vi "UI_Elmts_Reads[Labels].vi"(8 "error in (no error)":errorcluster, 10 "Elmts Labels":string[](array[string]), 11 "UI_Actor in":refnum<class "UI_Actor.lvclass">) -> (0 "error out":errorcluster, 1 "Founds":bool[](array[boolean]), 2 "Values":variant[](array[variant]), 3 "UI_Actor out":refnum<class "UI_Actor.lvclass">)   [LabVIEW 2020, in "UI_Actor.lvlib" / "UI_Actor.lvclass"]
uses:
  UI_Actor.lvclass
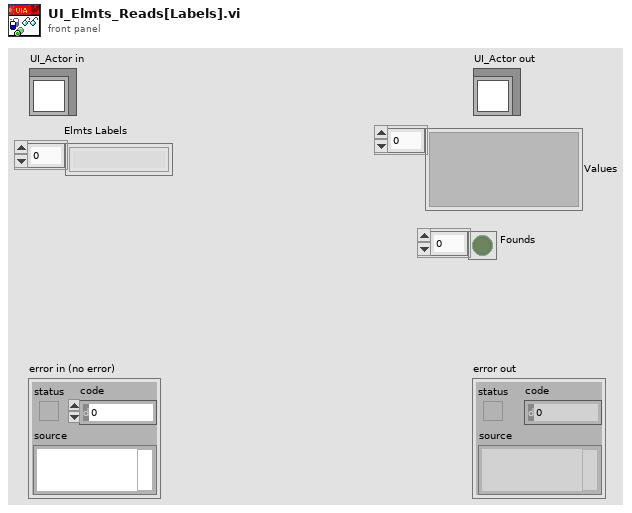
[diagram p1: front panel]
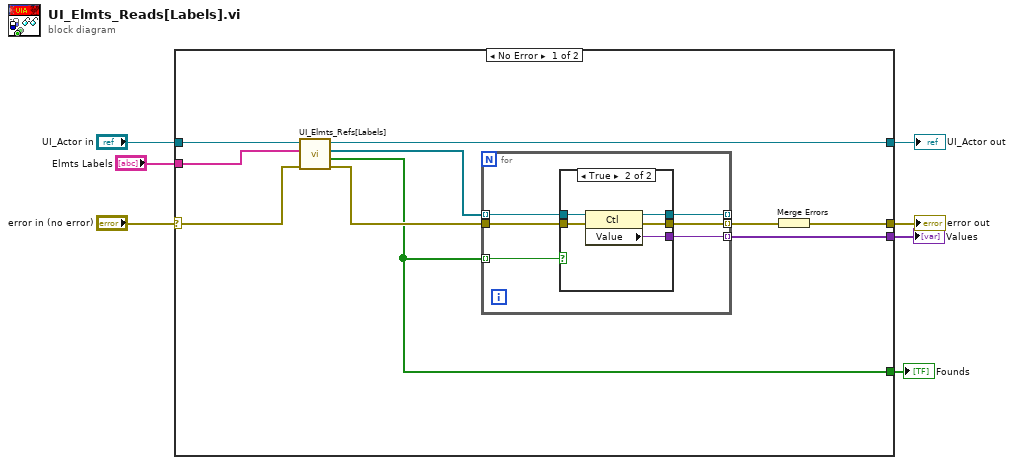
[diagram p0: block diagram]
diagram:
  n1 = case shown="No Error" "error in (no error)" {
    selector: "error in (no error)" -> [w12 w32]
    tunnel: [w14 w32] -> w6
    tunnel: [w16 w31] -> w4
    tunnel: "UI_Actor in" -> [w17 w31]
    tunnel: "Elmts Labels" -> [w15 _]
    tunnel: [w13 _] -> w1
    tunnel: [w8 _] -> w2
    frame No Error {
      n2 = call "UI_Elmts_Refs[Labels].vi"("error in (no error)"=w12, "Elmts Labels"=w15, "UI_Actor in"=w17) -> ("error out"=w11:errorcluster, "Founds"=w8:bool[], "Refs"=w10:refnum<vi>[], "UI_Actor out"=w16:refnum<class "UI_Actor.lvclass">)  [unwired: 5 in]
      n3 = for {
        tunnel: w10 -> [w21] mode=indexing
        tunnel: [w20] -> w13 mode=indexing
        tunnel: [w19] -> _ mode=indexing
        tunnel: w11 -> [w23]
        tunnel: [w22] -> w9 mode=indexing
        tunnel: w8 -> [w18] mode=indexing
        n4 = case shown="True" w18 {
          tunnel: w23 -> [w24 w30]
          tunnel: [w24 w29] -> w22
          tunnel: w21 -> [w25 w28]
          tunnel: [_ w27] -> w20
          tunnel: [w25 w26] -> w19
          frame False {
          }
          frame True {
            n5 = property class="Ctl"(reference=w28, error in=w30) -> (reference out=w26:refnum<vi>, error out=w29:errorcluster, "Value"=w27:variant)
          }
        }
      }
      n6 = Merge Errors(w9) -> (w14:errorcluster)
    }
    frame Error {
    }
  }
  "error out" <- w6
  "UI_Actor out" <- w4
  "Values" <- w1
  "Founds" <- w2
